vi "測定データ転記.vi"() -> ()   [LabVIEW 2021]
panel:
  out "測定転記一時データ":string[](array[string])
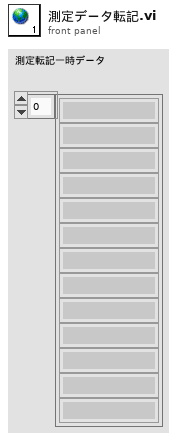
[diagram p1: front panel]
diagram:
